vi "bilineal.vi"(4 "input variable":dbl[][](array[numeric])) -> (1 "output variable":dbl[][](array[numeric]))   [LabVIEW 2018]
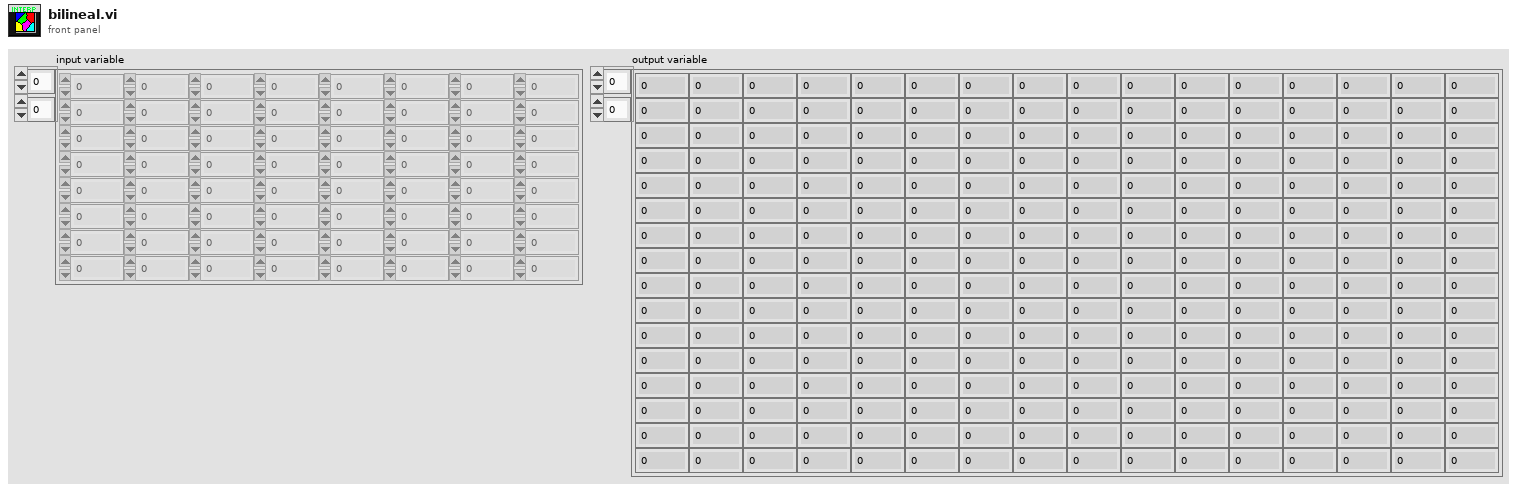
[diagram p1: front panel]
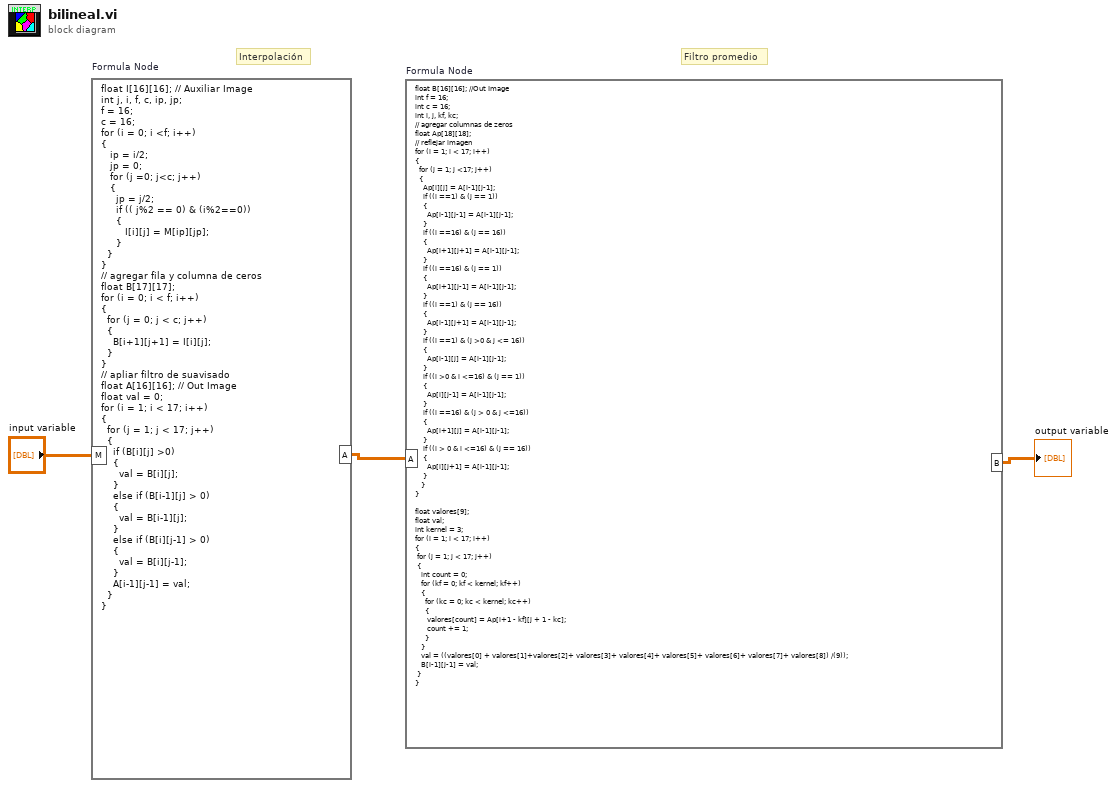
[diagram p0: block diagram]
diagram:
  # "Filtro promedio"
  # "Interpolación"
  n1 = formula code="float I[16][16]; // Auxiliar Image\nint j, i, f, c, ip, jp;\nf = 16;\nc = 16;\nfor (i = 0; i <f; i++)\n{\n   ip = i/2;\n   jp = 0;\n   for (j =0; j<c; j++)\n   {\n     jp = j/2;\n     if (( j%2 == 0) & (i%2==0))\n     {\n        I[i][j] = M[ip][jp];\n     }\n  }\n}\n// agregar fila y columna de ceros\nfloat B[17][17];\nfor (i = 0; i < f; i++)\n{\n  for (j = 0; j < c; j++)\n  { \n    B[i+1][j+1] = I[i][j];\n  }\n}\n// apliar filtro de suavisado\nfloat A[16][16]; // Out Image\nfloat val = 0;\nfor (i = 1; i < 17; i++)\n{\n  for (j = 1; j < 17; j++)\n  {\n    if (B[i][j] >0)\n    {\n      val = B[i][j];\n    }\n    else if (B[i-1][j] > 0)\n    {\n      val = B[i-1][j];\n    }\n    else if (B[i][j-1] > 0)\n    {\n      val = B[i][j-1];\n    }\n    A[i-1][j-1] = val;\n  }\n}"("M"="input variable") -> ("A"=w2:dbl[][])
  n2 = formula code="float B[16][16]; //Out Image\nint f = 16;\nint c = 16;\nint i, j, kf, kc;\n// agregar columnas de zeros\nfloat Ap[18][18];\n// reflejar imagen\nfor (i = 1; i < 17; i++)\n{\n  for (j = 1; j <17; j++)\n  {\n    Ap[i][j] = A[i-1][j-1];\n    if ((i ==1) & (j == 1))\n    {\n      Ap[i-1][j-1] = A[i-1][j-1];\n    }\n    if ((i ==16) & (j == 16))\n    {\n      Ap[i+1][j+1] = A[i-1][j-1];\n    }\n    if ((i ==16) & (j == 1))\n    {\n      Ap[i+1][j-1] = A[i-1][j-1];\n    }\n    if ((i ==1) & (j == 16))\n    {\n      Ap[i-1][j+1] = A[i-1][j-1];\n    }\n    if ((i ==1) & (j >0 & j <= 16))\n    {\n      Ap[i-1][j] = A[i-1][j-1];\n    }\n    if ((i >0 & i <=16) & (j == 1))\n    {\n      Ap[i][j-1] = A[i-1][j-1];\n    }\n    if ((i ==16) & (j > 0 & j <=16))\n    {\n      Ap[i+1][j] = A[i-1][j-1];\n    }\n    if ((i > 0 & i <=16) & (j == 16))\n    {\n      Ap[i][j+1] = A[i-1][j-1];\n    }\n   }\n} \n\nfloat valores[9];\nfloat val;\nint kernel = 3;\nfor (i = 1; i < 17; i++)\n{\n for (j = 1; j < 17; j++)\n {\n   int count = 0;\n   for (kf = 0; kf < kernel; kf++)\n   {\n     for (kc = 0; kc < kernel; kc++)\n     {\n      valores[count] = Ap[i+1 - kf][j + 1 - kc];\n      count += 1;\n     }\n   }\n   val = ((valores[0] + valores[1]+valores[2]+ valores[3]+ valores[4]+ valores[5]+ valores[6]+ valores[7]+ valores[8]) /(9));\n   B[i-1][j-1] = val;\n }\n}"("A"=w2) -> ("B"=→"output variable":dbl[][])
